vi "Move.vi"(3 "error in (no error)":errorcluster) -> (0 "error out":errorcluster, 1 "Turn":dbl, 2 "Forward":dbl)   [LabVIEW 2017]
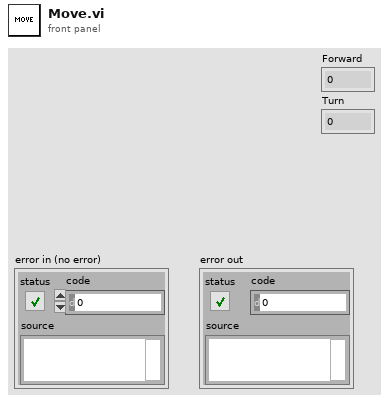
[diagram p1: front panel]
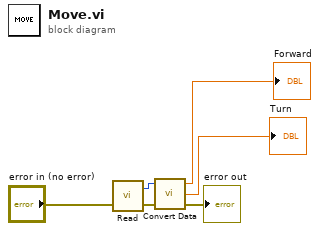
[diagram p0: block diagram]
diagram:
  n1 = call "Read.vi"("error in (no error)"="error in (no error)") -> ("error out"=w5:errorcluster, "Numeric Out"=w1:i16)  [unwired: 1 in]
  n2 = call "Convert Data.vi"("error in"=w5, "Data In"=w1) -> ("error out"=→"error out":errorcluster, "Turn"=→"Turn":dbl, "Forward"=→"Forward":dbl)  [unwired: 1 in]
